vi "App_Menu.vi"() -> ()   [LabVIEW 2015, in "Application 1.lvlib"]
uses:
  Application 1.lvlib
  Data Def/App_Subpanel Name.ctl
  Data Def/App_User Event Data.ctl
  Data Def/App_Tips Data.ctl
panel:
  in  "Monitor":bool
  in  "Query Data":bool
  in  "Training Mode":bool
  in  "User Setting":bool
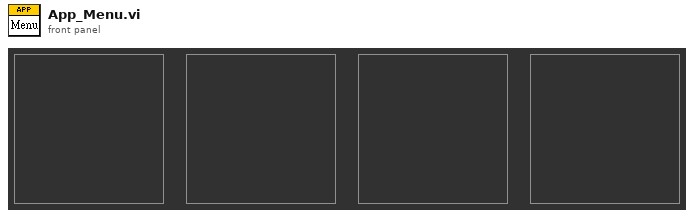
[diagram p1: front panel]
types:
  T1 = typedef "Application 1.lvlib/App_Tips Data.ctl" = cluster{"Tips":string, "BG Color":u32}
  T2 = typedef "Application 1.lvlib/App_User Event Data.ctl" = cluster{"Command":string, "Data":variant}
  T3 = typedef "Application 1.lvlib/App_Subpanel Name.ctl" = enum16{"Main", "Menu", "User Registering", "User Setting", "Monitor", "Traning Mode", "Query Data", "Connect Setting"}
  T4 = typedef "Application 1.lvlib/App_Main Data.ctl" = cluster{"VI Refnum":refnum<vi>, "Subpanel":refnum<vi>, "Connection ID":refnum<k5>, "Meta data":T5[], "Main Queue":T7, "User Data":T8}
  T5 = typedef "stm_MetaElement.ctl" = cluster{"Name":T6}
  T6 = typedef "stm_MetaDataElement.ctl" = string
  T7 = typedef "Application 1.lvlib/App_Main Queue.ctl" = cluster{"Main Loop Queue":refnum<queue>}
  T8 = typedef "User Data.ctl" = cluster{"Name":string, "Email":string, "Phone Number":string, "User Picture":u32[][], "Last Login Time":timestamp}
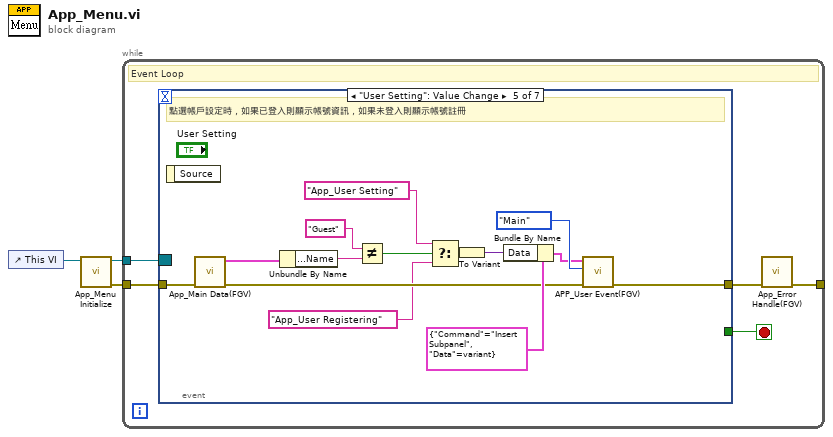
[diagram p0: block diagram]
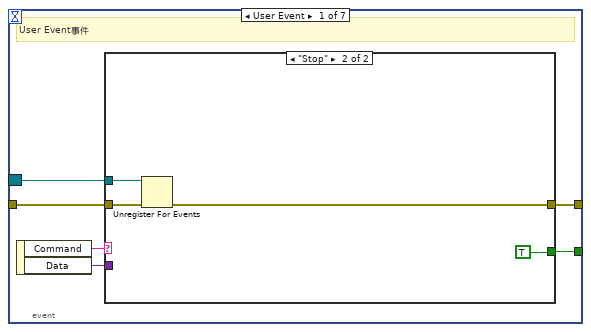
[diagram p2: hidden frame]
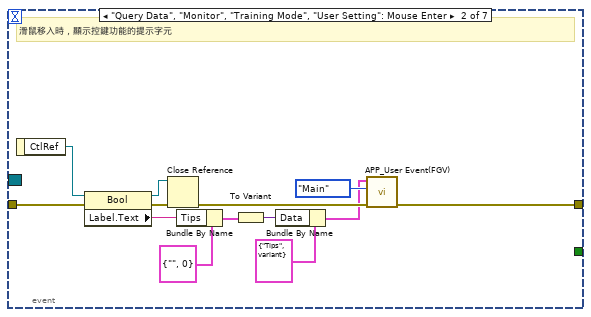
[diagram p4: hidden frame]
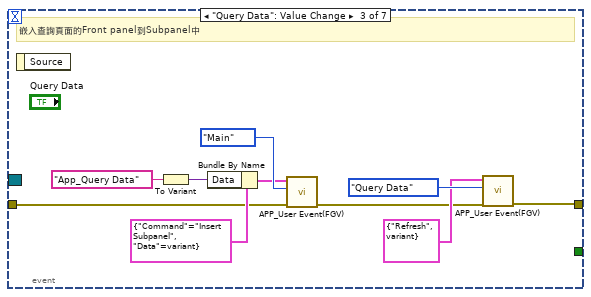
[diagram p5: hidden frame]
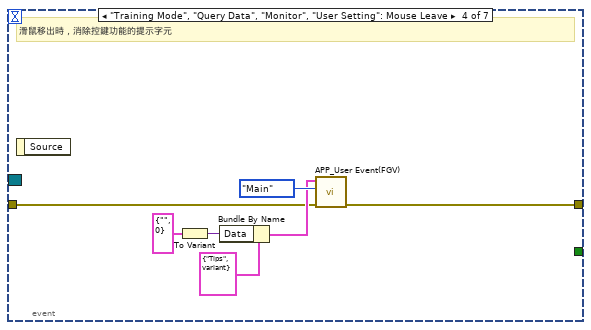
[diagram p6: hidden frame]
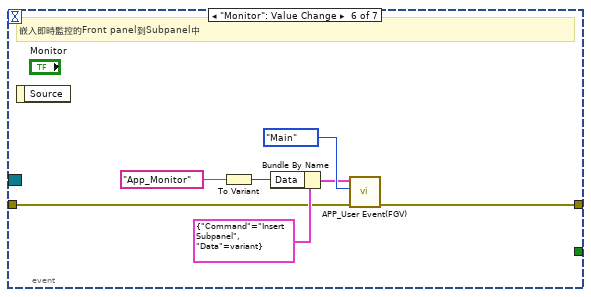
[diagram p7: hidden frame]
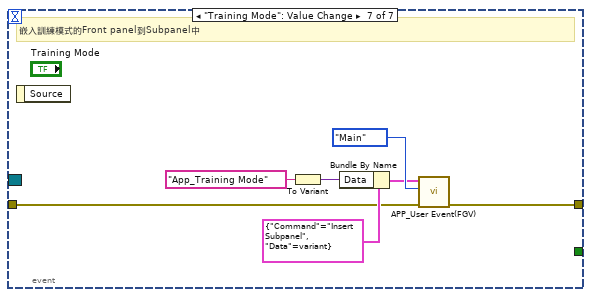
[diagram p8: hidden frame]
diagram:
  n1 = control-ref of="This VI"() -> (w3:refnum<vi>)
  n2 = call "App_Menu Initialize.vi"("VI Reference"=w3) -> ("error out"=w2:errorcluster, "Event Registration Refnum"=w1:refnum<event-registration>)  [unwired: 9 in]
  n3 = while {
    tunnel: w2 -> [w8]
    tunnel: w1 -> [w7]
    tunnel: [w5] -> _
    stop <- w4 stop-if-true
    # "Event Loop"
    n4 = event shown="[4] \"User Setting\": Value Change" {
      selector: w7 -> [w10 _ _ _ _ _ _]
      dyn-events: _ -> [_ _ _ _ _ _ _]
      timeout: _ -> [_ _ _ _ _ _ _]
      tunnel: w8 -> [w12 w32 w37 w45 w57 w66 w72]
      tunnel: [w11 w26 w33 w44 w59 w65 w71] -> w6
      tunnel: [w9 _ _ _ _ _ _] -> w4
      event User Event {
        # "User Event事件"
        n5 = event-data() -> ("Command"=w14:string, "Data"=w13:variant)  [unwired: 1 in]
        n6 = case shown="\"Stop\"" w14 {
          tunnel: w13 -> [_ _]
          tunnel: w12 -> [w15 w19]
          tunnel: [w15 w17] -> w11
          tunnel: w10 -> [_ w18]
          tunnel: [_ TRUE] -> w9
          frame Default {
          }
          frame "Stop" {
            n7 = Unregister For Events(event registration refnum=w18, error in=w19) -> (error out=w17:errorcluster)
          }
        }
      }
      event "Query Data", "Monitor", "Training Mode", "User Setting": Mouse Enter {
        # "滑鼠移入時，顯示控鍵功能的提示字元"
        n8 = event-data() -> ("CtlRef"=w31:refnum<vi>)  [unwired: 1 in]
        n9 = property class="Bool"(reference=w31, error in=w32) -> (reference out=w29:refnum<vi>, error out=w30:errorcluster, "Label.Text"=w21:string)
        n10 = Close Reference(reference=w29, error in (no error)=w30) -> (error out=w27:errorcluster)
        n11 = Bundle By Name(cluster=T1 {"Tips"="", "BG Color"=0} ("Tips Data"), "Tips"=w21) -> (w20:T1)
        n12 = To Variant(anything=w20) -> (Variant=w24:variant)
        n13 = Bundle By Name(cluster=T2 {"Command"="Tips", "Data"=variant} ("User Event Data"), "Data"=w24) -> (w23:T2)
        n14 = call "APP_User Event(FGV).vi"("error in"=w27, "Subpanel Name"=App_Subpanel_Name."Main", "User Event Data"=w23) -> ("error out"=w26:errorcluster)  [unwired: 7 in, 1 out]
      }
      event "Query Data": Value Change {
        # "嵌入查詢頁面的Front panel到Subpanel中"
        n15 = event-data() -> ()  [unwired: 1 in, 1 out]
        n16 = To Variant(anything="App_Query Data") -> (Variant=w41:variant)
        n17 = Bundle By Name(cluster=T2 {"Command"="Insert Subpanel", "Data"=variant} ("User Event Data"), "Data"=w41) -> (w39:T2)
        n18 = call "APP_User Event(FGV).vi"("error in"=w37, "Subpanel Name"=App_Subpanel_Name."Main", "User Event Data"=w39) -> ("error out"=w34:errorcluster)  [unwired: 7 in, 1 out]
        n19 = call "APP_User Event(FGV).vi"("error in"=w34, "Subpanel Name"=App_Subpanel_Name."Query Data", "User Event Data"=T2 {"Command"="Refresh", "Data"=variant}) -> ("error out"=w33:errorcluster)  [unwired: 7 in, 1 out]
      }
      event "Training Mode", "Query Data", "Monitor", "User Setting": Mouse Leave {
        # "滑鼠移出時，消除控鍵功能的提示字元"
        n20 = event-data() -> ()  [unwired: 1 in, 1 out]
        n21 = To Variant(anything=T1 {"Tips"="", "BG Color"=0} ("Tips Data")) -> (Variant=w47:variant)
        n22 = Bundle By Name(cluster=T2 {"Command"="Tips", "Data"=variant} ("User Event Data"), "Data"=w47) -> (w46:T2)
        n23 = call "APP_User Event(FGV).vi"("error in"=w45, "Subpanel Name"=App_Subpanel_Name."Main", "User Event Data"=w46) -> ("error out"=w44:errorcluster)  [unwired: 7 in, 1 out]
      }
      event "User Setting": Value Change {
        # "點選帳戶設定時，如果已登入則顯示帳號資訊，如果未登入則顯示帳號註冊"
        n24 = event-data() -> ()  [unwired: 1 in, 1 out]
        n25 = call "App_Main Data(FGV).vi"("error in"=w57) -> ("error out"=w56:errorcluster, "Main Data Out"=w55:T4)  [unwired: 9 in]
        n26 = Unbundle By Name(w55) -> ("User Data.Name"=w53:string)
        n27 = Not Equal?(x="Guest", y=w53) -> (x != y?=w52:bool)
        n28 = Select(t="App_User Setting", s=w52, f="App_User Registering") -> (s? t:f=w58:string)
        n29 = To Variant(anything=w58) -> (Variant=w62:variant)
        n30 = Bundle By Name(cluster=T2 {"Command"="Insert Subpanel", "Data"=variant} ("User Event Data"), "Data"=w62) -> (w60:T2)
        n31 = call "APP_User Event(FGV).vi"("error in"=w56, "Subpanel Name"=App_Subpanel_Name."Main", "User Event Data"=w60) -> ("error out"=w59:errorcluster)  [unwired: 7 in, 1 out]
      }
      event "Monitor": Value Change {
        # "嵌入即時監控的Front panel到Subpanel中"
        n32 = event-data() -> ()  [unwired: 1 in, 1 out]
        n33 = To Variant(anything="App_Monitor") -> (Variant=w69:variant)
        n34 = Bundle By Name(cluster=T2 {"Command"="Insert Subpanel", "Data"=variant} ("User Event Data"), "Data"=w69) -> (w67:T2)
        n35 = call "APP_User Event(FGV).vi"("error in"=w66, "Subpanel Name"=App_Subpanel_Name."Main", "User Event Data"=w67) -> ("error out"=w65:errorcluster)  [unwired: 7 in, 1 out]
      }
      event "Training Mode": Value Change {
        # "嵌入訓練模式的Front panel到Subpanel中"
        n36 = event-data() -> ()  [unwired: 1 in, 1 out]
        n37 = To Variant(anything="App_Training Mode") -> (Variant=w76:variant)
        n38 = Bundle By Name(cluster=T2 {"Command"="Insert Subpanel", "Data"=variant} ("User Event Data"), "Data"=w76) -> (w74:T2)
        n39 = call "APP_User Event(FGV).vi"("error in"=w72, "Subpanel Name"=App_Subpanel_Name."Main", "User Event Data"=w74) -> ("error out"=w71:errorcluster)  [unwired: 7 in, 1 out]
      }
    }
    n40 = call "App_Error Handle(FGV).vi"("error in"=w6) -> ("error out"=w5:errorcluster)  [unwired: 9 in, 1 out]
  }
